vi "readHeader.vi"(8 "error in (no error)":errorcluster, 11 "ModbusBuffer in":refnum<class "ModbusBufferBuilder.lvclass">) -> (0 "error out":errorcluster, 1 "Length":u16, 2 "Subnet":u8, 3 "ModbusBuffer out":refnum<class "ModbusBufferBuilder.lvclass">)   [LabVIEW 2016, in "ModbusBufferBuilder.lvclass"]
uses:
  ModbusBufferBuilder.lvclass
  ModbusBufferBuilder.lvclass/ModbusBufferBuilder.ctl
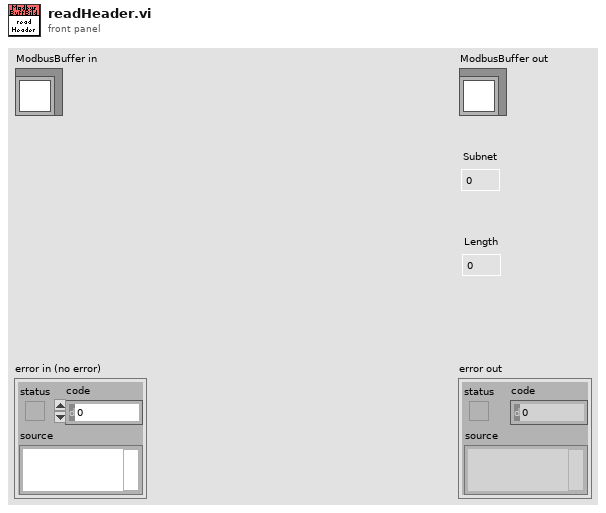
[diagram p1: front panel]
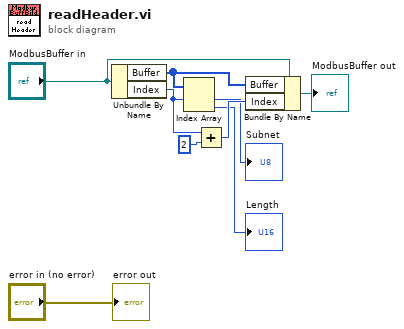
[diagram p0: block diagram]
diagram:
  n1 = Unbundle By Name("ModbusBuffer in") -> ("Buffer"=w8:u16[], "Index"=w7:i32)
  n2 = Index Array(array=w8, index #1=w7) -> (element #1=→"Subnet":u16, element #2=→"Length":u16)  [unwired: 1 in]
  n3 = Add(x=w7, y=2) -> (x+y=w5:i32)
  n4 = Bundle By Name(cluster="ModbusBuffer in", "Buffer"=w8, "Index"=w5) -> (→"ModbusBuffer out":refnum<class "ModbusBufferBuilder.lvclass">)
  "error out" <- "error in (no error)"
